vi "HDPE Fit VI window to Selected Decoration with option .vi"(6 "Object No":i32=1, 7 "Reference":enum16{"Top Left", "Bottom Right"}(ring), 8 "error in (no error)":errorcluster, 10 "Border Spacing":i16=2, 11 "VI Ref (calling VI)":refnum<vi>) -> (0 "error out":errorcluster, 3 "Dup VI Ref":refnum<vi>)   [LabVIEW 2019]
doc: "This utility will fit (resize and center) a VI (defined by the \"VI Ref\" input) about the given largest decoration in that VI. It will add a border defined by border spacing in units of pixels. If there are no decorations found in the VI it is a no-op and will not produce an error. Unfortunately, this VI can not find locked decorations (yet).\n\nUsage Caveat: If the caller VI's <B>Minimum Panel Size</B> is set to a size larger than the size of its largest decoration, this VI will give out an error.\n\nCopyright © 2011, Unilogic Technologies. All rights reserved."
uses:
  <vilib>/Utility/miscctls.llb/LVPointTypeDef.ctl
panel:
  in  "Case Constant\n(See Context Help)":bool
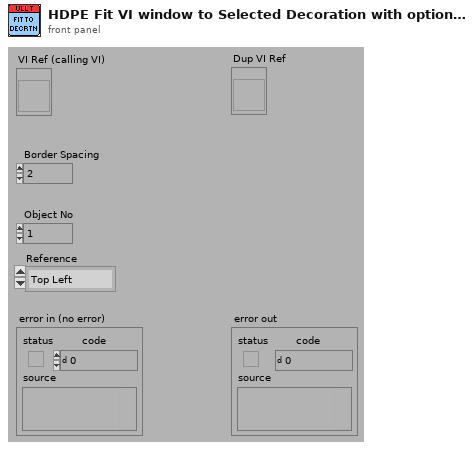
[diagram p1: front panel]
types:
  T1 = typedef "LVPointTypeDef.ctl" = cluster{"Horizontal":i16, "Vertical":i16}
  T2 = typedef "LVRectTypeDef.ctl" = cluster{"Left":i16, "Top":i16, "Right":i16, "Bottom":i16}
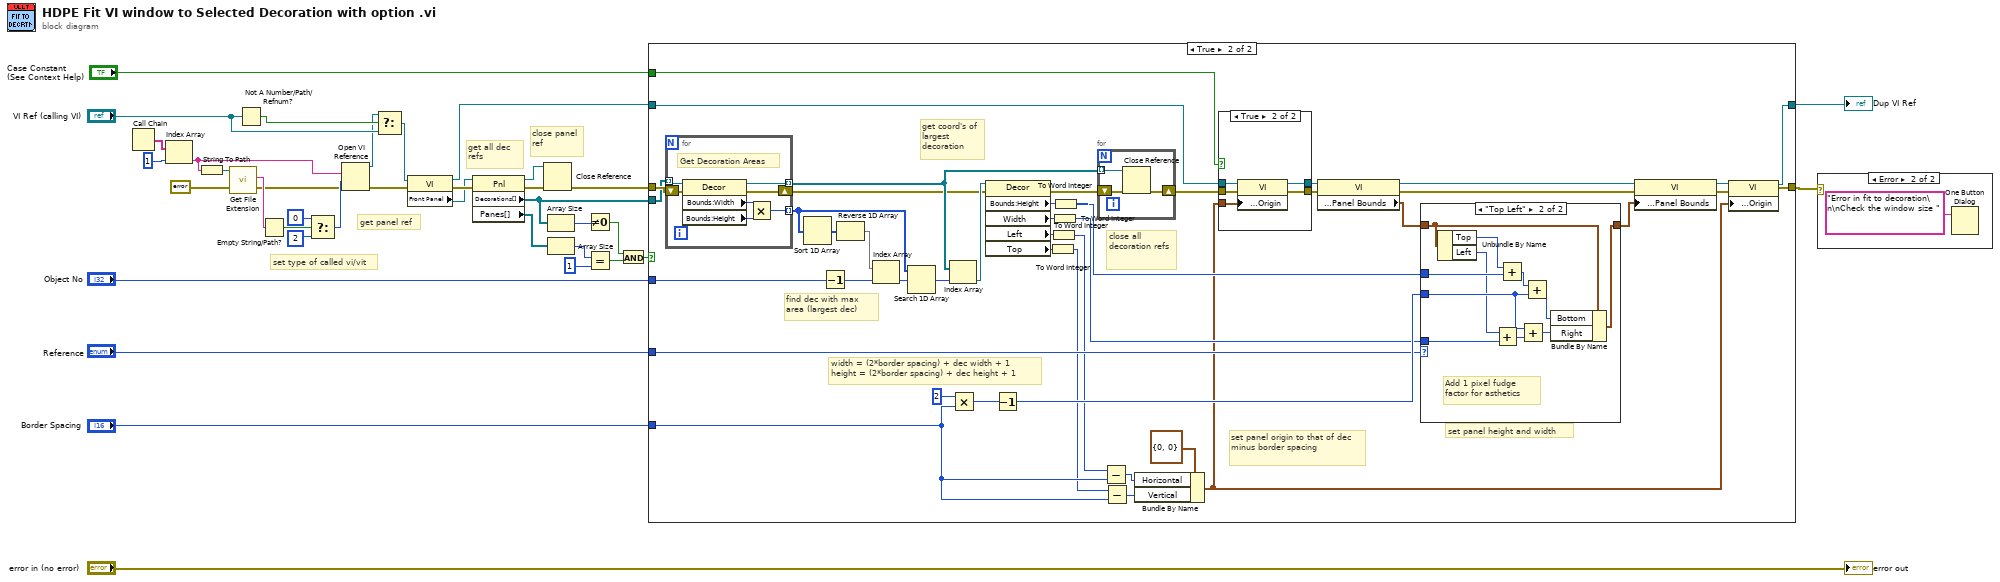
[diagram p0: block diagram]
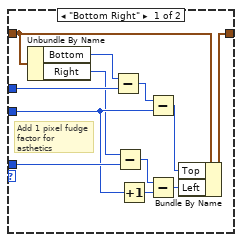
[diagram p3: hidden frame]
diagram:
  # "set type of called vi/vit"
  # "close panel ref"
  # "get all dec refs"
  # "get panel ref"
  n1 = Call Chain() -> (call chain=w26:string[])
  n2 = Index Array(array=w26, index=1 ("Index")) -> (element=w17:string)
  n3 = String To Path(string=w17) -> (path=w16:path)
  n4 = call <vilib>:"Get File Extension.vi"("error in (no error)"=errorcluster {"status"=FALSE, "code"=0, "source"=""} ("error IO"), "file"=w16) -> ("error out"=w9:errorcluster, "lowercase file extension"=w15:string)  [unwired: 5 in, 3 out]
  n5 = Not A Number/Path/Refnum?(number/path/refnum="VI Ref (calling VI)") -> (NaN/Path/Refnum?=w23:bool)
  n6 = Empty String/Path?(string/path=w15) -> (empty?=w14:bool)
  n7 = Select(t=0 ("options"), s=w14, f=2 ("options")) -> (s? t:f=w11:i32)
  n8 = Open VI Reference(vi path=w17, options=w11, error in (no error)=w9) -> (vi reference=w22:refnum<vi>, error out=w8:errorcluster)  [unwired: 3 in]
  n9 = Select(t=w22, s=w23, f="VI Ref (calling VI)") -> (s? t:f=w24:refnum<vi>)
  n10 = property on="Property Node" class="VI"(reference=w24, error in=w8) -> (reference out=w20:refnum<vi>, error out=w29:errorcluster, "Front Panel"=w18:refnum<vi>)
  n11 = property on="Property Node" class="Pnl"(reference=w18, error in=w29) -> (reference out=w19:refnum<vi>, error out=w28:errorcluster, "Decorations[]"=w21:refnum<vi>[], "Panes[]"=w7:refnum<vi>[])
  n12 = Close Reference(reference=w19, error in (no error)=w28) -> (error out=w27:errorcluster)
  n13 = Array Size(array=w21) -> (size(s)=w6:i32)
  n14 = Array Size(array=w7) -> (size(s)=w5:i32)
  n15 = Not Equal To 0?(x=w6) -> (x != 0?=w2:bool)
  n16 = Equal?(x=w5, y=1) -> (x = y?=w3:bool)
  n17 = And(x=w2, y=w3) -> (x .and. y?=w1:bool)
  n18 = case shown="True" w1 {
    tunnel: w27 -> [w39 w78]
    tunnel: [w39 w62] -> w35
    tunnel: [w38 w61] -> w36
    tunnel: w21 -> [_ w70]
    tunnel: "Object No" -> [_ w58]
    tunnel: "Reference" -> [_ w57]
    tunnel: w20 -> [w38 w50]
    tunnel: "Border Spacing" -> [_ w51]
    tunnel: "Case Constant\n(See Context Help)" -> [_ w45]
    frame False {
      # "do nothing if no decorations"
    }
    frame True {
      # "get coord's of largest decoration"
      # "close all  decoration refs"
      # "set panel height and width"
      # "set panel origin to that of dec minus border spacing"
      # "width = (2*border spacing) + dec width + 1\nheight = (2*border spacing) + dec height + 1"
      # "find dec with max area (largest dec)"
      n19 = for {
        tunnel: w70 -> [w119] mode=indexing
        tunnel: [w116] -> w66 mode=indexing
        shift-right: [w114] -> w75
        shift-left: w78 -> [w115]
        tunnel: [w113] -> w77 mode=indexing
        # "Get Decoration Areas"
        n20 = property class="Decor"(reference=w119, error in=w115) -> (reference out=w113:refnum<vi>, error out=w114:errorcluster, "Bounds:Width"=w118:u32, "Bounds:Height"=w117:u32)
        n21 = Multiply(x=w118, y=w117) -> (x*y=w116:u32)
      }
      n22 = Sort 1D Array(array=w66) -> (sorted array=w69:u32[])
      n23 = Decrement(x=w58) -> (x-1=w67:i32)
      n24 = Reverse 1D Array(array=w69) -> (reversed array=w68:u32[])
      n25 = Index Array(array=w68, index=w67) -> (element=w64:u32)
      n26 = Search 1D Array(1D array=w66, element=w64) -> (index of element=w65:i32)  [unwired: 1 in]
      n27 = Index Array(array=w77, index=w65) -> (element=w76:refnum<vi>)
      n28 = Multiply(x=i16 2 ("y"), y=w51) -> (x*y=w60:i16)
      n29 = property class="Decor"(reference=w76, error in=w75) -> (error out=w74:errorcluster, "Bounds:Height"=w80:u32, "Width"=w56:u32, "Left"=w53:i32, "Top"=w52:i32)  [unwired: 1 out]
      n30 = Decrement(x=w60) -> (x-1=w59:i16)
      n31 = To Word Integer(number=w52) -> (16bit integer=w48:i16)
      n32 = To Word Integer(number=w53) -> (16bit integer=w49:i16)
      n33 = To Word Integer(number=w56) -> (16bit integer=w46:i16)
      n34 = To Word Integer(number=w80) -> (16bit integer=w47:i16)
      n35 = for {
        tunnel: w77 -> [w122] mode=indexing
        shift-right: [w120] -> w72
        shift-left: w74 -> [w121]
        n36 = Close Reference(reference=w122, error in (no error)=w121) -> (error out=w120:errorcluster)
      }
      n37 = Subtract(x=w49, y=w51) -> (x-y=w43:i16)
      n38 = Subtract(x=w48, y=w51) -> (x-y=w44:i16)
      n39 = Bundle By Name(cluster=T1 {"Horizontal"=0, "Vertical"=0} ("Front Panel Window:Origin"), "Horizontal"=w43, "Vertical"=w44) -> (w41:T1)
      n40 = case shown="True" w45 {
        tunnel: [w106 w112] -> w82
        tunnel: w50 -> [w106 w111]
        tunnel: w41 -> [_ w108]
        tunnel: w72 -> [w107 w110]
        tunnel: [w107 w109] -> w71
        frame False {
        }
        frame True {
          n41 = property on="Property Node" class="VI"(reference=w111, error in=w110, "Front Panel Window:Origin"=w108) -> (reference out=w112:refnum<vi>, error out=w109:errorcluster)
        }
      }
      n42 = property on="Property Node" class="VI"(reference=w82, error in=w71) -> (reference out=w42:refnum<vi>, error out=w40:errorcluster, "Front Panel Window:Panel Bounds"=w79:T2)
      n43 = case shown="\"Top Left\"" w57 {
        tunnel: [w90 w101] -> w81
        tunnel: w46 -> [w89 w97]
        tunnel: w47 -> [w88 w100]
        tunnel: w79 -> [w86 w98]
        tunnel: w59 -> [w85 w96]
        frame "Bottom Right" {
          # "Add 1 pixel fudge factor for asthetics"
          n44 = Unbundle By Name(w86) -> ("Bottom"=w87:i16, "Right"=w83:i16)
          n45 = Subtract(x=w87, y=w88) -> (x-y=w93:i16)
          n46 = Subtract(x=w83, y=w89) -> (x-y=w91:i16)
          n47 = Increment(x=w85) -> (x+1=w84:i16)
          n48 = Subtract(x=w93, y=w85) -> (x-y=w94:i16)
          n49 = Subtract(x=w91, y=w84) -> (x-y=w92:i16)
          n50 = Bundle By Name(cluster=w86, "Top"=w94, "Left"=w92) -> (w90:T2)
        }
        frame "Top Left" {
          # "Add 1 pixel fudge factor for asthetics"
          n51 = Unbundle By Name(w98) -> ("Top"=w99:i16, "Left"=w95:i16)
          n52 = Add(x=w95, y=w97) -> (x+y=w102:i16)
          n53 = Add(x=w99, y=w100) -> (x+y=w104:i16)
          n54 = Add(x=w96, y=w102) -> (x+y=w103:i16)
          n55 = Add(x=w104, y=w96) -> (x+y=w105:i16)
          n56 = Bundle By Name(cluster=w98, "Bottom"=w105, "Right"=w103) -> (w101:T2)
        }
      }
      n57 = property on="Property Node" class="VI"(reference=w42, error in=w40, "Front Panel Window:Panel Bounds"=w81) -> (reference out=w63:refnum<vi>, error out=w55:errorcluster)
      n58 = property on="Property Node" class="VI"(reference=w63, error in=w55, "Front Panel Window:Origin"=w41) -> (reference out=w61:refnum<vi>, error out=w62:errorcluster)
    }
  }
  "Dup VI Ref" <- w36
  n59 = case shown="Error" w35 {
    frame No Error {
    }
    frame Error {
      n60 = One Button Dialog(message="Error in fit to decoration\n\nCheck the window size ") -> ()  [unwired: 1 in, 1 out]
    }
  }
  "error out" <- "error in (no error)"
